vi "Stop Core.vi"(10 "final error code":i32, 11 "GUI Container Actor in":refnum<class "GUI Container Actor.lvclass">) -> (3 "GUI Container Actor out":refnum<class "GUI Container Actor.lvclass">)   [LabVIEW 2023, in "GUI Views.lvlib" / "GUI Container Actor.lvclass"]
doc: "In addition to the following, this method also sends a message to the monitor to notify it that the actor has stopped execution.\n\n(<B>Filename</B>: Actor Framework.lvlib:Actor.lvclass:Stop Core.vi)\n\nDefines what the actor does before it stops. Use the <B>final error code</B> input to determine whether the actor shut down in response to an error.\n\nBy default, this method does nothing. A descendant class may override it to define behavior, such as shutting down any processes the actor initiated in its override of the Actor Core method.\n\nCopyright: MGI\n\nAuthored by Derek Trepanier\nsupport@mooregoodideas.com\nwww.mooregoodideas.com\n\nCopyright (c) 2014, Moore Good Ideas, Inc.\n\nAll rights reserved.\n\nRedistribution and use in source and binary forms, with or without modification, are permitted provided that the following conditions are met:\n\n * Redistributions of source code must retain the above copyright notice, this list of conditions and the following disclaimer.\n * Redistributions in binary form must reproduce the above copyright notice, this list of conditions and the following disclaimer in the documentation and/or other materials provided with the distribution.\n * Neither the name of Moore Good Ideas, Inc. nor the names of its contributors may be used to endorse or promote products derived from this software without specific prior written permission.\n\nTHIS SOFTWARE IS PROVIDED BY THE COPYRIGHT HOLDERS AND CONTRIBUTORS \"AS IS\" AND ANY EXPRESS OR IMPLIED WARRANTIES, INCLUDING, BUT NOT LIMITED TO, THE IMPLIED WARRANTIES OF MERCHANTABILITY AND FITNESS FOR A PARTICULAR PURPOSE ARE DISCLAIMED. IN NO EVENT SHALL THE COPYRIGHT OWNER OR CONTRIBUTORS BE LIABLE FOR ANY DIRECT, INDIRECT, INCIDENTAL, SPECIAL, EXEMPLARY, OR CONSEQUENTIAL DAMAGES (INCLUDING, BUT NOT LIMITED TO, PROCUREMENT OF SUBSTITUTE GOODS OR SERVICES; LOSS OF USE, DATA, OR PROFITS; OR BUSINESS INTERRUPTION) HOWEVER CAUSED AND ON ANY THEORY OF LIABILITY, WHETHER IN CONTRACT, STRICT LIABILITY, OR TORT (INCLUDING NEGLIGENCE OR OTHERWISE) ARISING IN ANY WAY OUT OF THE USE OF THIS SOFTWARE, EVEN IF ADVISED OF THE POSSIBILITY OF SUCH DAMAGE."
uses:
  GUI Container Actor.lvclass
  GUI Container Actor.lvclass/GUI Container Actor.ctl
  GUI View Actor/GUI View Actor.lvclass
  <userlib>/_OpenG.lib/error/error.llb/openg_error.lvlib
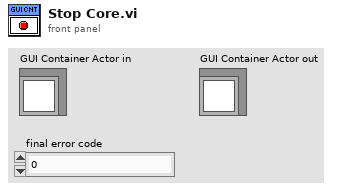
[diagram p1: front panel]
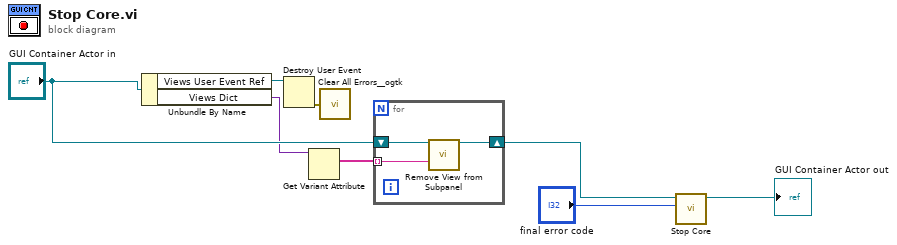
[diagram p0: block diagram]
diagram:
  n1 = Unbundle By Name("GUI Container Actor in") -> ("Views User Event Ref"=w6:refnum<user-event>, "Views Dict"=w2:variant)
  n2 = Destroy User Event(user event=w6) -> (error out=w5:errorcluster)  [unwired: 1 in]
  n3 = Get Variant Attribute(Variant=w2) -> (names=w3:string[])  [unwired: 3 in, 3 out]
  n4 = call <userlib>:"Clear All Errors__ogtk.vi"("Error In"=w5) -> ()  [unwired: 3 in, 1 out]
  n5 = for {
    tunnel: w3 -> [w11] mode=indexing
    shift-right: [w9] -> w1
    shift-left: "GUI Container Actor in" -> [w10]
    n6 = call "Remove View from Subpanel.vi"("GUI Container Actor in"=w10, "Subpanel"=w11) -> ("GUI Container Actor out"=w9:refnum<class "GUI Container Actor.lvclass">)  [unwired: 12 in, 1 out]
  }
  n7 = call-parent "Stop Core.vi"("final error code"="final error code", "GUI View Actor in"=w1) -> ("GUI View Actor out"=→"GUI Container Actor out":refnum<class "GUI Container Actor.lvclass">)  [unwired: 9 in]
